vi "GetOperatingState.vi"(8 "error in":errorcluster, 9 "op state":string, 10 "operating states":variant, 11 "data group":string) -> (0 "error out":errorcluster, 3 "operating state":T1)   [LabVIEW 2017, in "Trigger.lvlib"]
uses:
  <vilib>/addons/InsightCM/Devices/Shared/Common/Trigger/Trigger.lvlib
  <vilib>/addons/InsightCM/Devices/Shared/Common/Trigger/controls/TriggerOperatingState.ctl
  <vilib>/addons/InsightCM/MessageBus/Base/controls/KeyValuePair.ctl
  <vilib>/addons/InsightCM/Devices/Shared/Common/Trigger/controls/TriggerCondition.ctl
  <vilib>/addons/InsightCM/MessageBus/Base/controls/Condition.ctl
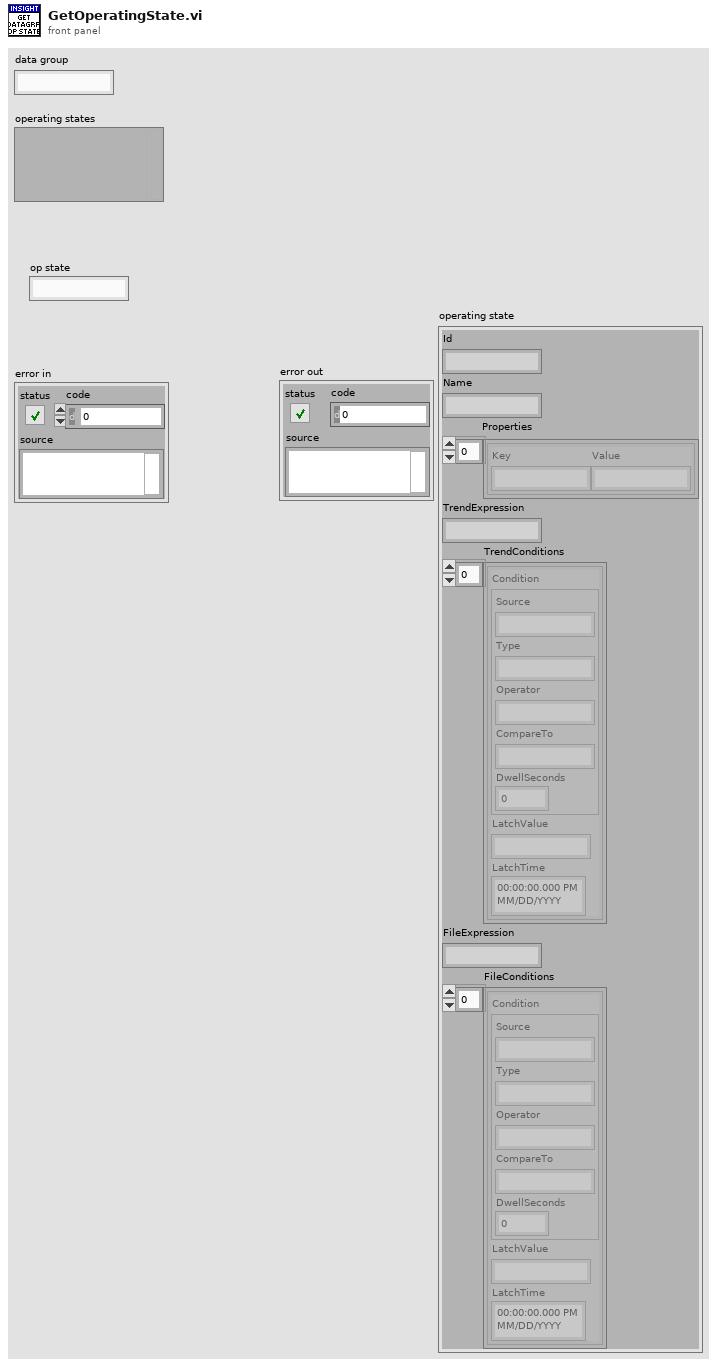
[diagram p1: front panel]
types:
  T1 = typedef "Trigger.lvlib/TriggerOperatingState.ctl" = cluster{"Id":string, "Name":string, "Properties":T2[], "TrendExpression":string, "TrendConditions":T3[], "FileExpression":string, "FileConditions":T3[]}
  T2 = typedef "KeyValuePair.ctl" = cluster{"Key":string, "Value":string}
  T3 = typedef "Trigger.lvlib/TriggerCondition.ctl" = cluster{"Condition":T4, "LatchValue":string, "LatchTime":timestamp}
  T4 = typedef "Condition.ctl" = cluster{"Source":string, "Type":string, "Operator":string, "CompareTo":string, "DwellSeconds":dbl}
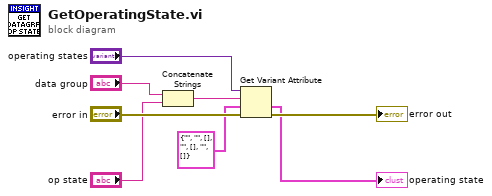
[diagram p0: block diagram]
diagram:
  n1 = Concatenate Strings("data group", "op state") -> (w3:string)
  n2 = Get Variant Attribute(Variant="operating states", name=w3, default value (empty Variant)=T1 {"Id"="", "Name"="", "Properties"=[], "TrendExpression"="", "TrendConditions"=[], "FileExpression"="", "FileConditions"=[]} ("OperatingState"), error in="error in") -> (value=→"operating state":T1, error out=→"error out":errorcluster)  [unwired: 2 out]
